vi "Main.vi"(8 "error in":errorcluster, 11 "ChartView Worker in":refnum<class "ChartView Worker.lvclass">) -> (0 "error out":errorcluster, 3 "ChartView Worker out":refnum<class "ChartView Worker.lvclass">)   [LabVIEW 2018, in "ChartView Worker.lvclass"]
doc: "The Queued Message Handler of a Worker."
uses:
  ChartView Worker.lvclass
  D:/Program Files (x86)/National Instruments/LabVIEW 2018/vi.lib/addons/_Workers/Library/Classes/Worker/Worker.lvclass
  <vilib>/addons/_Workers/Library/Classes/Worker/Worker.lvclass/Worker.ctl
  Initialization Data.ctl
  <vilib>/addons/_Workers/Library/Classes/Message Queue/Message Queue.lvclass
  ChartView Worker.lvclass/ChartView Worker.ctl
  <vilib>/addons/_Workers/Library/Classes/Worker/Read Alias.vi
  <vilib>/addons/_Workers/Library/Classes/Message/Enqueue Message to Queue.vi
  <vilib>/addons/_Workers/Library/Classes/Worker/Worker.lvclass
  <vilib>/addons/_Workers/Library/Classes/Message/Message.lvclass
  Acquire Worker/DataAcquire Worker.lvclass
  D:/Program Files (x86)/National Instruments/LabVIEW 2018/vi.lib/addons/_Workers/Library/Classes/Workers Object/Workers Object.lvclass
panel:
  out "字符串":string
  out "波形图表":dbl(graph)
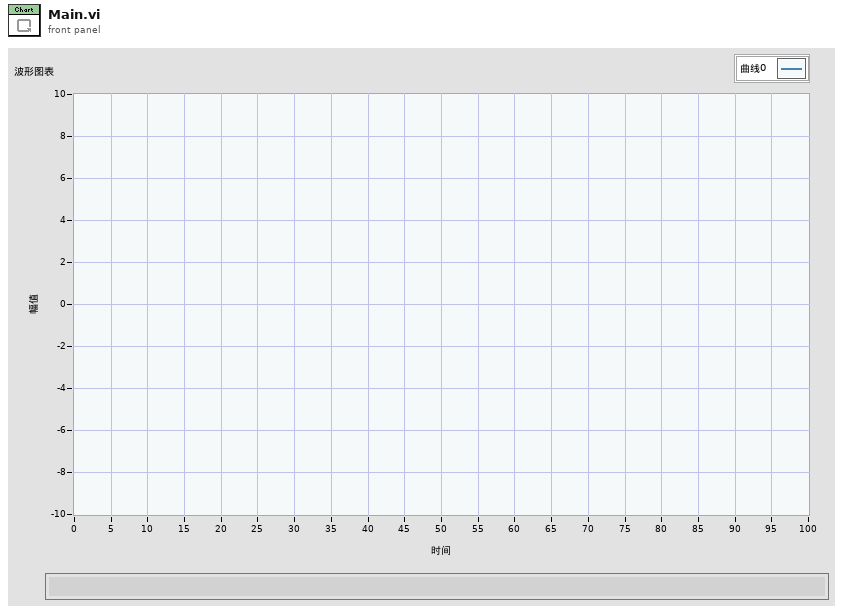
[diagram p1: front panel]
types:
  T1 = typedef "ChartView Worker.lvclass/Initialization Data.ctl" = cluster{"String":string, "Acquire Queue":refnum<class "Message Queue.lvclass">}
  T2 = typedef "Workers.lvlib/Case Label.ctl" = string
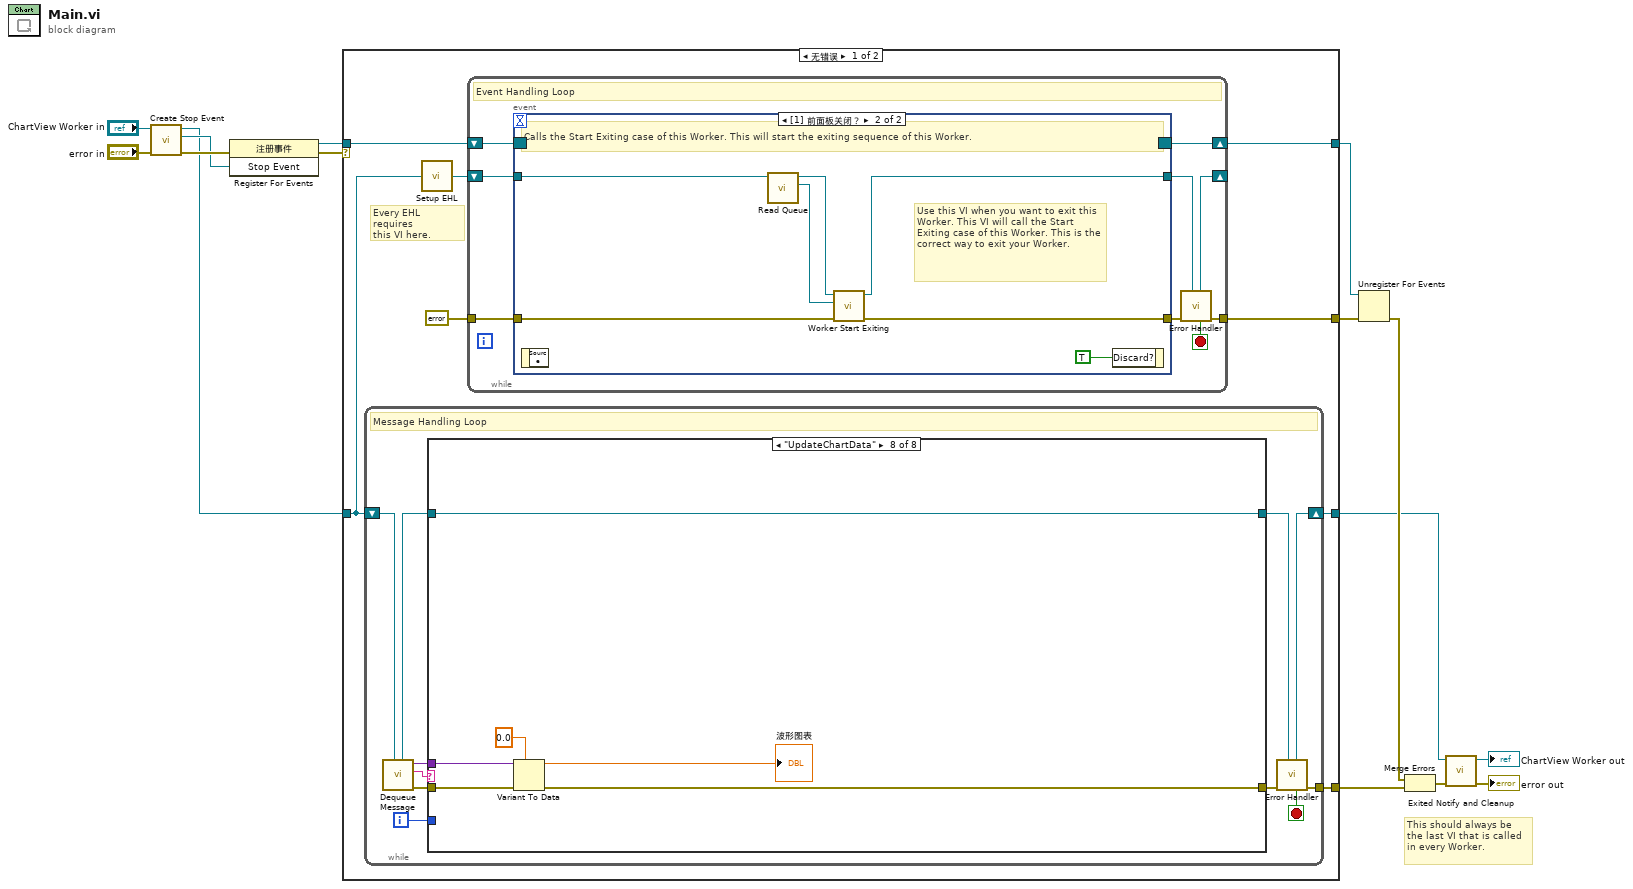
[diagram p0: block diagram]
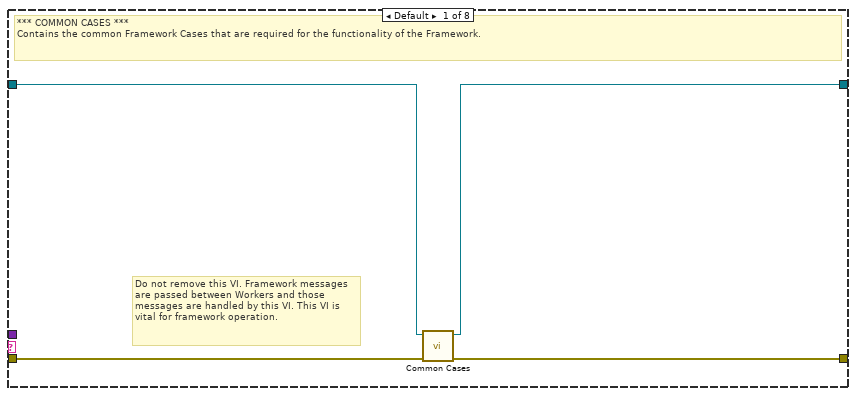
[diagram p2: hidden frame]
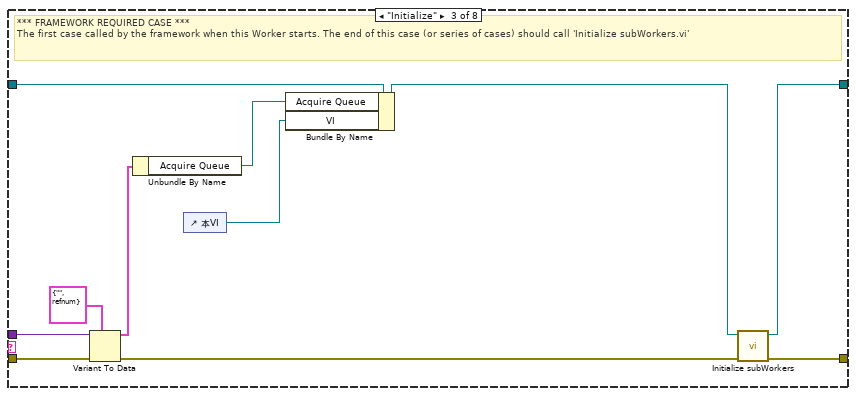
[diagram p4: hidden frame]
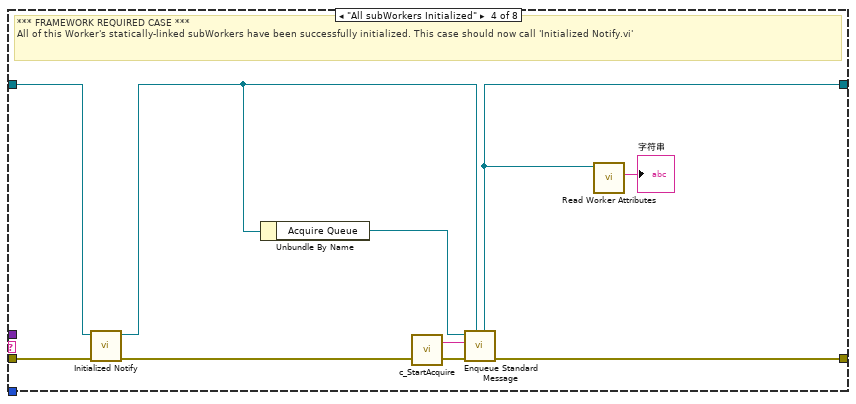
[diagram p5: hidden frame]
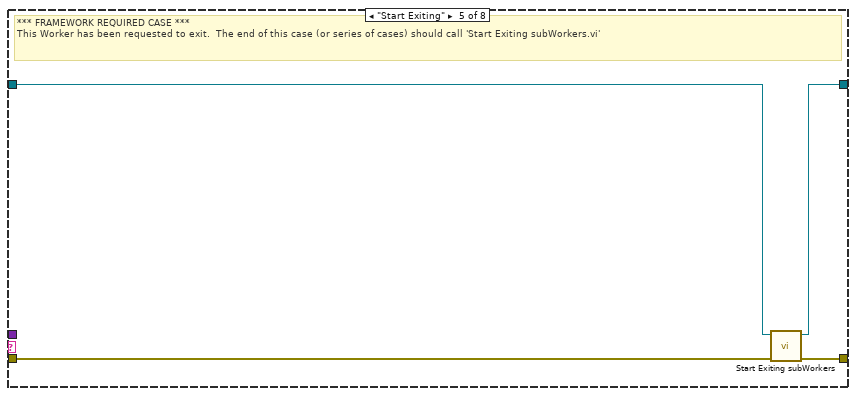
[diagram p6: hidden frame]
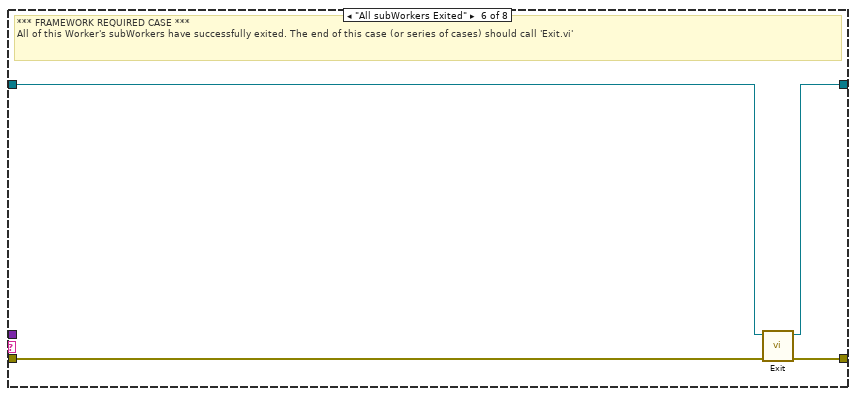
[diagram p7: hidden frame]
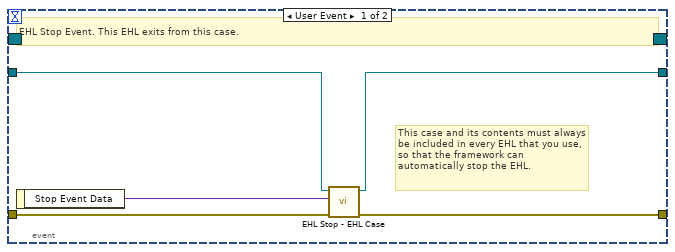
[diagram p9: hidden frame]
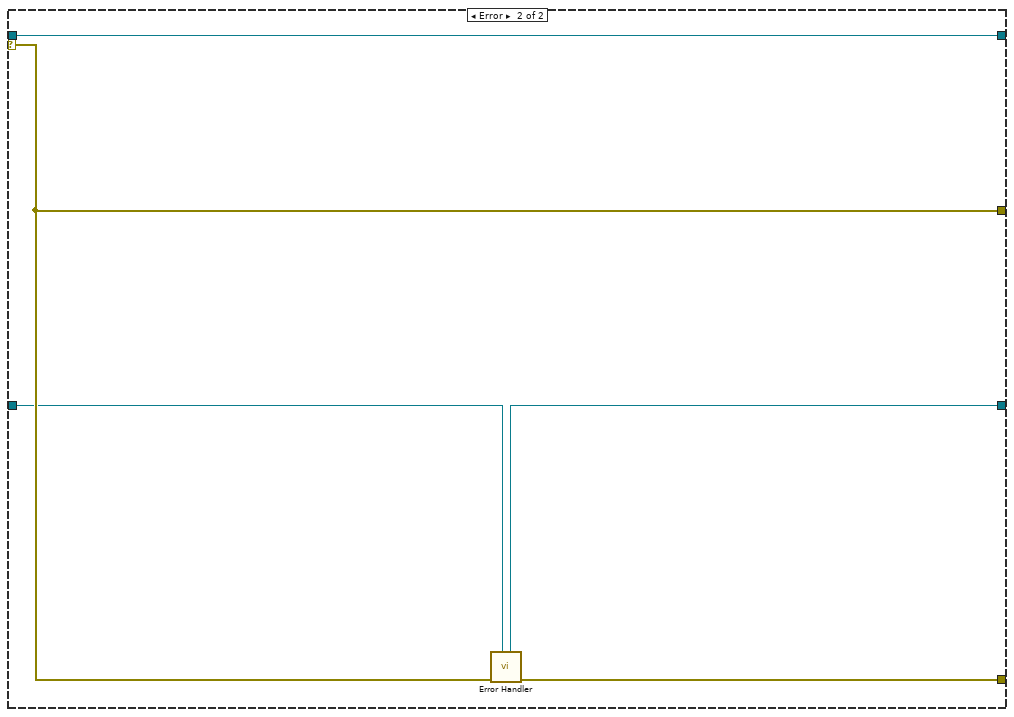
[diagram p10: hidden frame]
diagram:
  # "This should always be the last VI that is called in every Worker."
  n1 = call-dynamic "Create Stop Event.vi"("error in"="error in", "Worker"="ChartView Worker in") -> ("error out"=w10:errorcluster, "Stop Event"=w7:refnum<user-event>, "Worker out"=w4:refnum<class "ChartView Worker.lvclass">)  [unwired: 7 in]
  n2 = register-events(error in=w10, w7) -> (reference out=w9:refnum<event-registration>, error out=w1:errorcluster)  [unwired: 1 in]
  n3 = case shown="无错误" w1 {
    tunnel: w4 -> [w18 w99]
    tunnel: [w16 w100] -> w8
    tunnel: w9 -> [w23 w101]
    tunnel: [w20 w102] -> w14
    tunnel: [w22 w101] -> w13
    tunnel: [w17 w98] -> w11
    selector: w1 -> [_ w102]
    frame No Error {
      # "Every EHL requires\nthis VI here."
      n4 = while {
        shift-right: [w32] -> w17
        shift-left: w18 -> [w34]
        tunnel: [w33] -> w16
        i -> [w24]
        stop <- w25 stop-if-true
        # "Message Handling Loop"
        n5 = call-dynamic "Dequeue Message.vi"("Worker"=w34) -> ("error out"=w31:errorcluster, "Case out"=w26:string, "Data out"=w27:variant, "Worker out"=w29:refnum<class "ChartView Worker.lvclass">)  [unwired: 6 in, 1 out]
        n6 = case "Worker MHL Case Structure (DO NOT CHANGE LABEL NAME)" shown="\"UpdateChartData\"" w26 {
          tunnel: w31 -> [w38 w39 w49 w59 w61 w68 w69 w73]
          tunnel: [w37 w39 w51 w56 w64 w67 w69 w72] -> w30
          tunnel: w29 -> [w36 w40 w48 w60 w62 w66 w70 w76]
          tunnel: [w35 w40 w50 w55 w63 w65 w70 w76] -> w28
          tunnel: w27 -> [_ _ w46 _ _ _ _ w75]
          tunnel: w24 -> [_ _ _ _ _ _ _ _]
          frame Default {
            # "Do not remove this VI. Framework messages are passed between Workers and those messages are handled by this VI. This VI is vital for framework operation."
            # "*** COMMON CASES ***\nContains the common Framework Cases that are required for the functionality of the Framework."
            n7 = call-dynamic "Common Cases.vi"("error in"=w38, "Comm Worker in"=w36) -> ("error out"=w37:errorcluster, "Comm Worker out"=w35:refnum<class "ChartView Worker.lvclass">)  [unwired: 8 in]
          }
          frame "------ FRAMEWORK REQUIRED CASES ------" {
            # "Start of Framework Required Cases"
          }
          frame "Initialize" {
            # "*** FRAMEWORK REQUIRED CASE ***\nThe first case called by the framework when this Worker starts. The end of this case (or series of cases) should call 'Initialize subWorkers.vi'"
            n8 = Variant To Data(error in=w49, type=T1 {"String"="", "Acquire Queue"=refnum} ("Initialization Data"), Variant=w46) -> (data=w44:T1, error out=w47:errorcluster)
            n9 = Unbundle By Name(w44) -> ("Acquire Queue"=w42:refnum<class "Message Queue.lvclass">)
            n10 = control-ref of="本VI"() -> (w41:refnum<vi>)
            n11 = Bundle By Name(cluster=w48, "Acquire Queue"=w42, "VI"=w41) -> (w43:refnum<class "ChartView Worker.lvclass">)
            n12 = call-dynamic "Initialize subWorkers.vi"("error in"=w47, "Worker"=w43) -> ("error out"=w51:errorcluster, "dup Worker out"=w50:refnum<class "ChartView Worker.lvclass">)  [unwired: 8 in]
          }
          frame "All subWorkers Initialized" {
            # "*** FRAMEWORK REQUIRED CASE ***\nAll of this Worker's statically-linked subWorkers have been successfully initialized. This case should now call 'Initialized Notify.vi'"
            n13 = call-dynamic "Initialized Notify.vi"("error in"=w59, "Worker"=w60) -> ("error out"=w58:errorcluster, "dup Worker out"=w53:refnum<class "ChartView Worker.lvclass">)  [unwired: 8 in]
            n14 = Unbundle By Name(w53) -> ("Acquire Queue"=w52:refnum<class "Message Queue.lvclass">)
            n15 = call "c_StartAcquire.vi"() -> ("Case Label"=w54:T2)  [unwired: 1 in]
            n16 = call-poly <vilib>:"Enqueue Standard Message.vi"("Worker"=w53, "error in"=w58, "Case Label"=w54, "Message Queue"=w52) -> ("error out"=w56:errorcluster, "dup Worker out"=w55:refnum<class "ChartView Worker.lvclass">)  [unwired: 5 in, 1 out]
            n17 = call-poly <vilib>:"Read Worker Attributes.vi"("Worker"=w55) -> ("Alias out"=→"字符串":string)  [unwired: 9 in, 1 out]
          }
          frame "Start Exiting" {
            # "*** FRAMEWORK REQUIRED CASE ***\nThis Worker has been requested to exit.  The end of this case (or series of cases) should call 'Start Exiting subWorkers.vi'"
            n18 = call-dynamic "Start Exiting subWorkers.vi"("error_in"=w61, "Worker"=w62) -> ("error out"=w64:errorcluster, "dup Worker out"=w63:refnum<class "ChartView Worker.lvclass">)  [unwired: 8 in]
          }
          frame "All subWorkers Exited" {
            # "*** FRAMEWORK REQUIRED CASE ***\nAll of this Worker's subWorkers have successfully exited. The end of this case (or series of cases) should call 'Exit.vi'"
            n19 = call-dynamic "Exit.vi"("error_in"=w68, "Worker"=w66) -> ("error out"=w67:errorcluster, "dup Worker out"=w65:refnum<class "ChartView Worker.lvclass">)  [unwired: 8 in]
          }
          frame "-----------------------------------------------" {
            # "End of Framework Required Cases"
          }
          frame "UpdateChartData" {
            n20 = Variant To Data(error in=w73, type=0.0, Variant=w75) -> (data=→"波形图表":dbl, error out=w72:errorcluster)
          }
        }
        n21 = call-dynamic "Error Handler.vi"("Worker"=w28, "error_in"=w30) -> ("error out"=w33:errorcluster, "Stop Loop"=w25:bool, "Worker out"=w32:refnum<class "ChartView Worker.lvclass">)  [unwired: 7 in]
      }
      n22 = call-dynamic "Setup EHL.vi"("Worker"=w18) -> ("Worker out"=w19:refnum<class "ChartView Worker.lvclass">)  [unwired: 14 in]
      n23 = while "Event Handling Loop" {
        shift-right: [w85] -> w22
        shift-left: w23 -> [w84]
        tunnel: [w80] -> w20
        tunnel: errorcluster {"status"=FALSE, "code"=0, "source"=""} ("error constant") -> [w82]
        shift-right: [w78] -> _
        shift-left: w19 -> [w83]
        stop <- w77 stop-if-true
        # "Event Handling Loop"
        n24 = event shown="[1] 前面板关闭？" {
          selector: w84 -> [_ _]
          dyn-events: [_ _] -> w85
          timeout: _ -> [_ _]
          tunnel: [w89 w96] -> w81
          tunnel: w82 -> [w90 w95]
          tunnel: w83 -> [w88 w94]
          tunnel: [w87 w93] -> w79
          event User Event {
            # "This case and its contents must always be included in every EHL that you use, so that the framework can automatically stop the EHL."
            # "EHL Stop Event. This EHL exits from this case."
            n25 = event-data() -> ("Stop Event Data"=w86:variant)  [unwired: 1 in]
            n26 = call <vilib>:"EHL Stop - EHL Case.vi"("error in"=w90, "Stop Event Data"=w86, "Worker"=w88) -> ("error out"=w89:errorcluster, "Worker out"=w87:refnum<class "ChartView Worker.lvclass">)  [unwired: 7 in]
          }
          event Panel Close? {
            # "Use this VI when you want to exit this Worker. This VI will call the Start Exiting case of this Worker. This is the correct way to exit your Worker."
            # "Calls the Start Exiting case of this Worker. This will start the exiting sequence of this Worker."
            n27 = event-data() -> ()  [unwired: 1 in, 1 out]
            n28 = call <vilib>:"Read Queue.vi"("Worker"=w94) -> ("Message Queue out"=w91:refnum<class "Message Queue.lvclass">, "dup Worker out"=w92:refnum<class "ChartView Worker.lvclass">)  [unwired: 9 in]
            n29 = call-dynamic "Worker Start Exiting.vi"("error_in"=w95, "Message Queue"=w91, "Worker"=w92) -> ("error out"=w96:errorcluster, "dup Worker out"=w93:refnum<class "ChartView Worker.lvclass">)  [unwired: 7 in]
            n30 = event-data("Discard?"=TRUE) -> ()  [unwired: 1 in, 1 out]
          }
        }
        n31 = call-dynamic "Error Handler.vi"("Worker"=w79, "error_in"=w81) -> ("error out"=w80:errorcluster, "Stop Loop"=w77:bool, "Worker out"=w78:refnum<class "ChartView Worker.lvclass">)  [unwired: 7 in]
      }
    }
    frame Error {
      n32 = call-dynamic "Error Handler.vi"("Worker"=w99, "error_in"=w102) -> ("error out"=w100:errorcluster, "Worker out"=w98:refnum<class "ChartView Worker.lvclass">)  [unwired: 7 in, 1 out]
    }
  }
  n33 = Unregister For Events(event registration refnum=w13, error in=w14) -> (error out=w15:errorcluster)
  n34 = Merge Errors(w15, w8) -> (w12:errorcluster)
  n35 = call-dynamic "Exited Notify and Cleanup.vi"("error_in"=w12, "Worker"=w11) -> ("error out"=→"error out":errorcluster, "dup Worker out"=→"ChartView Worker out":refnum<class "ChartView Worker.lvclass">)  [unwired: 8 in]
